vi "Header Exists.vi"(8 "error in (no error)":errorcluster, 10 "header":string(combo)="User-Agent", 11 "HTTP Client Advanced in":refnum<class "HTTP Client Advanced.lvclass">) -> (0 "error out":errorcluster, 1 "value":string, 2 "header exists?":bool, 3 "HTTP Client Advanced out":refnum<class "HTTP Client Advanced.lvclass">)   [LabVIEW 2021, in "HTTP Client Advanced.lvclass"]
uses:
  HTTP Client Advanced.lvclass
  HTTP Client Advanced.lvclass/HTTP Client Advanced.ctl
  <vilib>/NI/Advanced HTTP Client/Session.lvclass
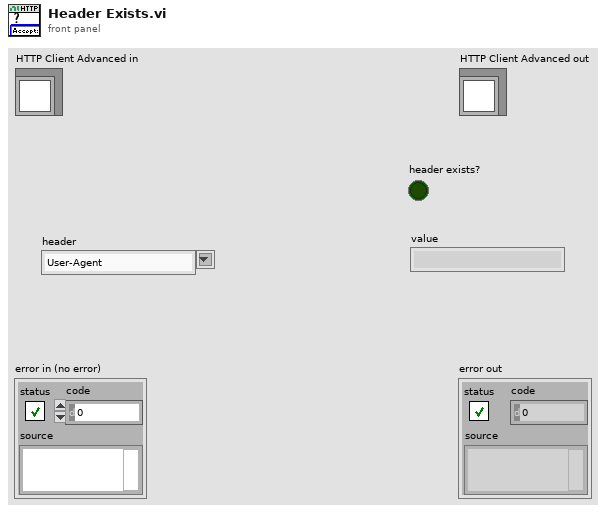
[diagram p1: front panel]
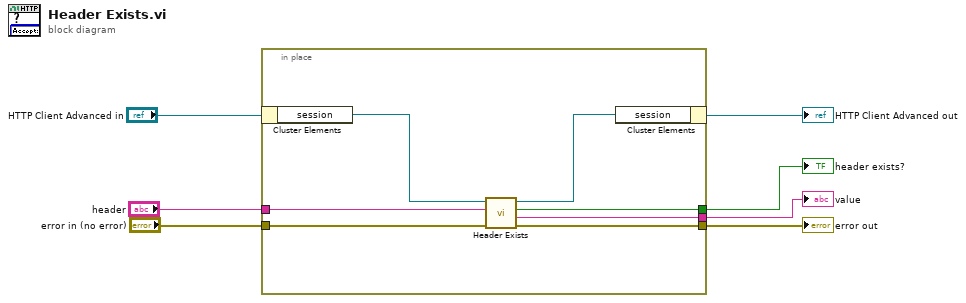
[diagram p0: block diagram]
diagram:
  n1 = in-place {
    in-place-border: "error in (no error)" -> [w14]
    in-place-border: [w13] -> w6
    in-place-border: "header" -> [w10]
    in-place-border: [w9] -> w2
    in-place-border: [w8] -> w1
    n2 = in-place-cluster #1("HTTP Client Advanced in") -> ("session"=w12:refnum<class "Session.lvclass">)
    n3 = call <vilib>:"Header Exists.vi"("error in"=w14, "header"=w10, "session in"=w12) -> ("error out"=w13:errorcluster, "value"=w9:string, "header exists?"=w8:bool, "session out"=w11:refnum<class "Session.lvclass">)  [unwired: 5 in]
    n4 = in-place-cluster #1("session"=w11) -> (→"HTTP Client Advanced out":refnum<class "HTTP Client Advanced.lvclass">)
  }
  "error out" <- w6
  "header exists?" <- w1
  "value" <- w2
